vi "LWXPS_GetJogVelocity.vi"(0 "XPS Reference IN":refnum<k24>, 11 "LabVIEW error IN":errorcluster) -> (3 "XPS Reference OUT":refnum<k24>, 4 "Returned error code":i32, 6 "Joystick Ack Timeout in ms":i32, 8 "Velocity X":dbl, 10 "Velocity Y":dbl, 14 "LabVIEW error OUT":errorcluster, 15 "XPS Error String":string)   [LabVIEW 2014]
uses:
  D:/XPSQ8_LabView_Library/Development/Source/Dll/Newport.XPS.CommandInterface.dll
  Dll/Newport.XPS.CommandInterface.dll
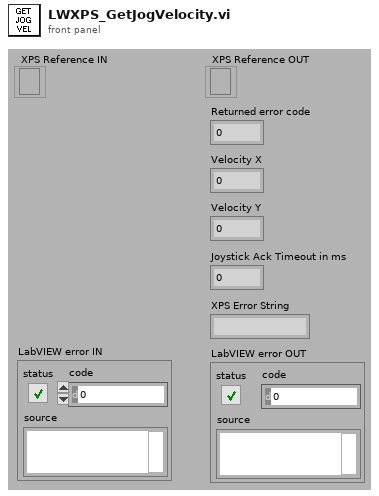
[diagram p1: front panel]
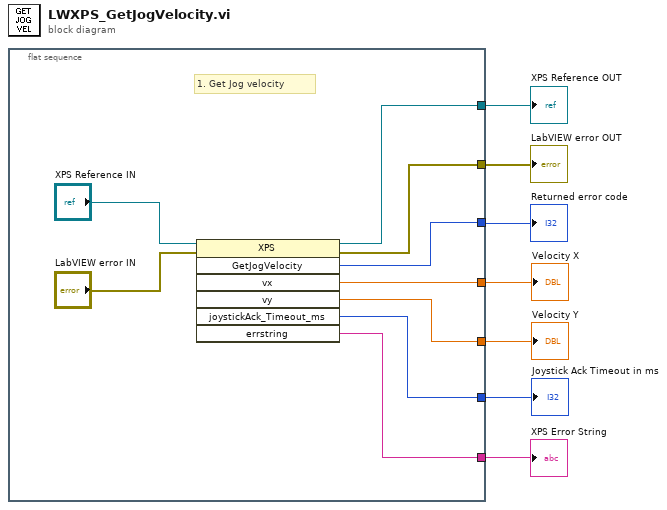
[diagram p0: block diagram]
diagram:
  n1 = flat-sequence {
    tunnel: [w15] -> w7
    tunnel: [w14] -> w6
    tunnel: [w13] -> w5
    tunnel: [w11] -> w3
    tunnel: [w10] -> w2
    tunnel: [w9] -> w1
    tunnel: [w8] -> w4
    frame #0 {
      # "1. Get Jog velocity"
      n2 = invoke class="XPS" method="GetJogVelocity"(reference="XPS Reference IN", error in="LabVIEW error IN") -> (reference out=w15:refnum<k24>, error out=w14:errorcluster, "GetJogVelocity"=w13:i32, "vx"=w11:dbl, "vy"=w10:dbl, "joystickAck_Timeout_ms"=w9:i32, "errstring"=w8:string)  [unwired: 5 in]
    }
  }
  "XPS Reference OUT" <- w7
  "LabVIEW error OUT" <- w6
  "Returned error code" <- w5
  "XPS Error String" <- w4
  "Velocity X" <- w3
  "Velocity Y" <- w2
  "Joystick Ack Timeout in ms" <- w1
